vi "SolarPanelSoftware_testeDigiRead.vi"() -> ()   [LabVIEW 2021]
uses:
  <vilib>/MakerHub/LINX/Public/Peripherals/Analog/Analog Read N Chans.vi
  <vilib>/MakerHub/LINX/Private/Local IO/LinxAnalogRead.vi
  <vilib>/MakerHub/LINX/Public/Utilities/Check Channel.vi
  <vilib>/MakerHub/LINX/Public/Utilities/Open Serial.vi
  <vilib>/MakerHub/LINX/Private/Utilties/Generate Error.vi
  <vilib>/MakerHub/LINX/Public/Sensors/Motion/Servo/Servo Open N Channels.vi
  <vilib>/MakerHub/LINX/Public/Sensors/Motion/Servo/Servo Set Pulse Width N Channels.vi
  <vilib>/MakerHub/LINX/Public/Sensors/Motion/Servo/Servo Close N Channels.vi
  <vilib>/MakerHub/LINX/LMH-LINX.lvlib
  <vilib>/MakerHub/LINX/Public/Sensors/Motion/Servo/Servo.lvlib
panel:
  in  "Start Button":bool
  out "BAIXO > CIMA":bool
  out "CIMA > BAIXO":bool
  out "DIR > ESQ":bool
  out "ESQ > DIR":bool
  in  "Servo Channels":i32[](array[numeric])=[9, 110]
  out "Angle Y":dbl
  in  "Threshold":dbl min=0.0 max=2.0 step=0.1
  out "Angle X":dbl
  out "Waveform Chart":T1(graph)
  out "Voltages":dbl[](array[numeric])
  in  "AI Channel(s)":u8[](array[numeric])
  in  "Stop Button":bool
  out "Loop Rate (Hz)":u32
  in  "Serial Port":refnum<visa-resource-name>
  out "ON":bool
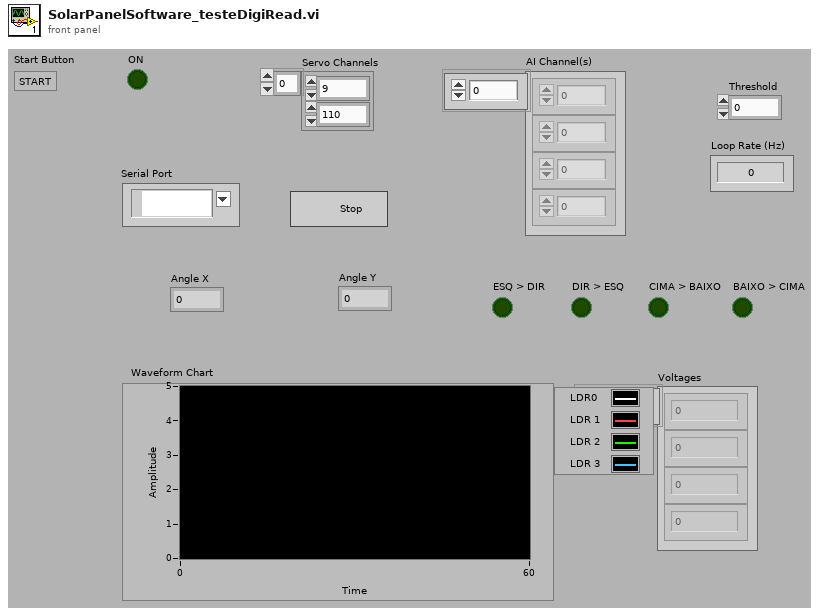
[diagram p1: front panel]
types:
  T1 = cluster{"Voltages[0]":dbl, "Voltages[1]":dbl, "Voltages[2]":dbl, "Voltages[3]":dbl, "Voltages[4]":dbl, "Voltages[5]":dbl, "Voltages[6]":dbl, "Voltages[7]":dbl, "Voltages[8]":dbl}
  T2 = typedef "LMH-LINX.lvlib/LINX Ref.ctl" = cluster{"IO":T3, "Interface":T4, "LINX Device Config":T5}
  T3 = typedef "LMH-LINX.lvlib/Platform.ctl" = enum16{"Remote", "Local"}
  T4 = typedef "LMH-LINX.lvlib/Interface.ctl" = enum16{"Serial", "TCP"}
  T5 = typedef "LMH-LINX.lvlib/Device.lvlib/LINX Device Config.ctl" = cluster{"Interface":T4, "COM Port":refnum<visa-resource-name>, "TCP Configuration":T6, "Device Family":u8, "Device ID":u8, "Device Name":string, "TCP Ref":refnum<k5>, "Channels":T7}
  T6 = typedef "LMH-LINX.lvlib/Device.lvlib/TCP Config.ctl" = cluster{"IP Address":string, "Port":u16}
  T7 = typedef "LMH-LINX.lvlib/Channels.ctl" = cluster{"DI":u8[], "DO":u8[], "AI":u8[], "AO":u8[], "PWM":u8[], "QE":u8[], "UART":u8[], "I2C 2":u8[], "SPI":u8[], "CAN":u8[], "Servo":u8[], "AI Ref (V)":dbl, "AI Resolution (Bits)":u8, "AO Ref (V)":dbl, "AO Resolution (Bits)":u8}
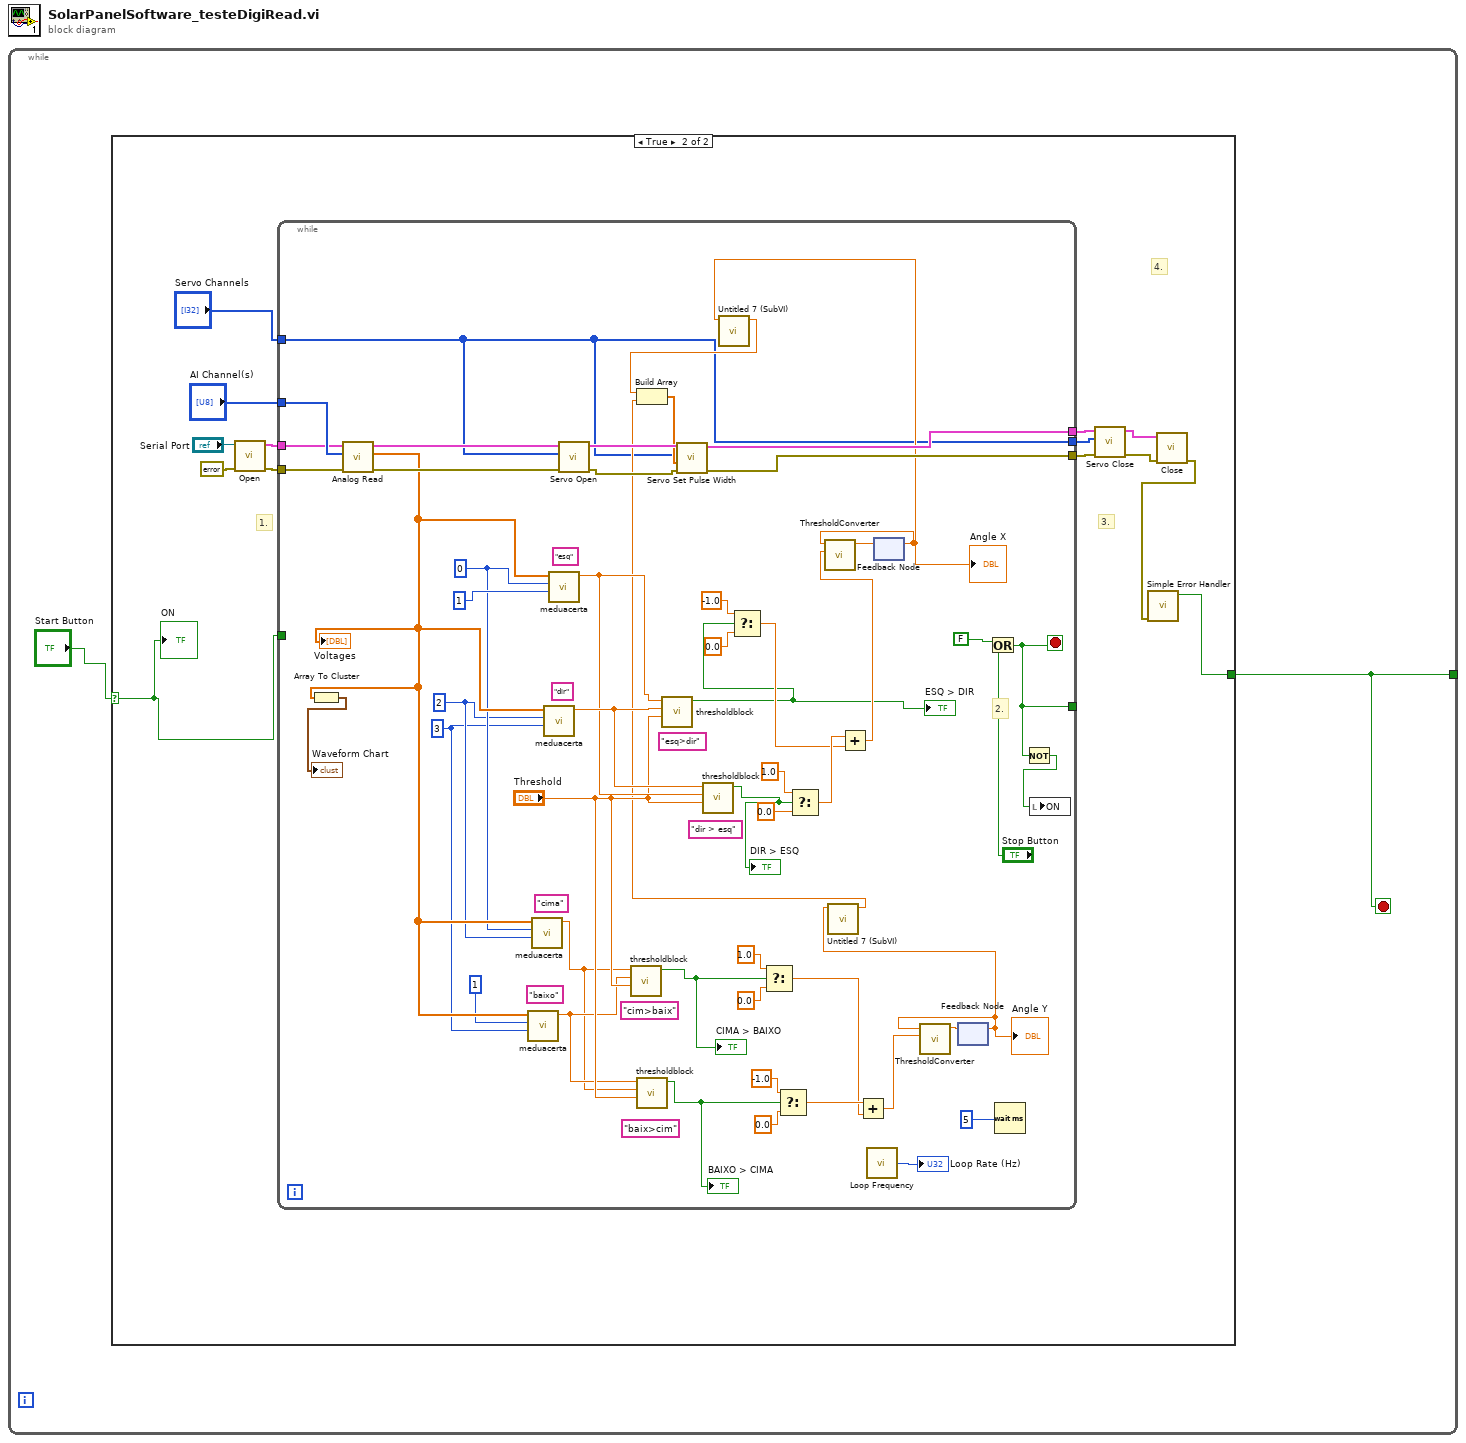
[diagram p0: block diagram]
diagram:
  n1 = while {
    tunnel: [w2] -> _
    stop <- w2 stop-if-true
    n2 = case shown="True" "Start Button" {
      selector: "Start Button" -> [w3 w6]
      tunnel: [w3 w5] -> w2
      frame False {
      }
      frame True {
        # "4."
        # "3."
        # "1."
        n3 = call-poly <vilib>:"Open.vi"("Error In"=errorcluster {"status"=FALSE, "code"=0, "source"=""}, "Serial Port"="Serial Port") -> ("Error Out"=w7:errorcluster, "LINX Resource"=w15:T2)  [unwired: 7 in, 1 out]
        n4 = while {
          tunnel: w15 -> [w66]
          tunnel: "AI Channel(s)" -> [w68]
          tunnel: [w19] -> _
          tunnel: "Servo Channels" -> [w20]
          tunnel: [w61] -> w13
          tunnel: [w60] -> w12
          tunnel: w7 -> [w58]
          tunnel: w6 -> [_]
          tunnel: [w20] -> w4
          stop <- w19 stop-if-true
          (unwired) "baix>cim" ("String")
          (unwired) "cim>baix" ("String")
          (unwired) "esq>dir" ("String")
          (unwired) "dir > esq" ("String")
          (unwired) "dir" ("String")
          (unwired) "esq" ("String")
          (unwired) "cima" ("String")
          (unwired) "baixo" ("String")
          w47 = 3 ("index")
          w49 = 2 ("index")
          w50 = 0 ("index")
          # "2."
          n5 = call-poly <vilib>:"Analog Read.vi"("Error In"=w58, "AI Channel(s)"=w68, "LINX Resource"=w66) -> ("Error Out"=w64:errorcluster, "Voltages"=w52:dbl[], "LINX Resource"=w65:T2)  [unwired: 5 in, 1 out]
          "Voltages" <- w52
          n6 = Array To Cluster(array=w52) -> (cluster=→"Waveform Chart":T1)
          n7 = call "meduacerta.vi"("index 1"=w47, "index 0"=1 ("index"), "Array"=w52) -> ("Média"=w36:dbl)  [unwired: 8 in]
          n8 = call "meduacerta.vi"("index 1"=w49, "index 0"=w50, "Array"=w52) -> ("Média"=w35:dbl)  [unwired: 8 in]
          n9 = call "meduacerta.vi"("index 1"=w47, "index 0"=w49, "Array"=w52) -> ("Média"=w46:dbl)  [unwired: 8 in]
          n10 = call "meduacerta.vi"("index 1"=1 ("index"), "index 0"=w50, "Array"=w52) -> ("Média"=w45:dbl)  [unwired: 8 in]
          n11 = call-poly <vilib>:"Servo Open.vi"("Error In"=w64, "Servo Channels"=w20, "LINX Resource"=w65) -> ("Error Out"=w63:errorcluster, "LINX Resource"=w62:T2)  [unwired: 7 in]
          n12 = call "thresholdblock.vi"("Threshold"="Threshold", "Média 2"=w36, "Média 1"=w35) -> ("Boolean"=w22:bool)  [unwired: 8 in]
          "CIMA > BAIXO" <- w22
          n13 = call "thresholdblock.vi"("Threshold"="Threshold", "Média 2"=w35, "Média 1"=w36) -> ("Boolean"=w21:bool)  [unwired: 8 in]
          "BAIXO > CIMA" <- w21
          n14 = call "thresholdblock.vi"("Threshold"="Threshold", "Média 2"=w46, "Média 1"=w45) -> ("Boolean"=w24:bool)  [unwired: 8 in]
          "ESQ > DIR" <- w24
          n15 = call "thresholdblock.vi"("Threshold"="Threshold", "Média 2"=w45, "Média 1"=w46) -> ("Boolean"=w23:bool)  [unwired: 8 in]
          "DIR > ESQ" <- w23
          n16 = Select(t=-1.0, s=w24, f=0.0) -> (s? t:f=w41:dbl)
          n17 = Select(t=1.0, s=w22, f=0.0) -> (s? t:f=w31:dbl)
          n18 = Select(t=-1.0, s=w21, f=0.0) -> (s? t:f=w32:dbl)
          n19 = Select(t=1.0, s=w23, f=0.0) -> (s? t:f=w42:dbl)
          n20 = Add(x=w42, y=w41) -> (x+y=w40:dbl)
          n21 = Add(x=w32, y=w31) -> (x+y=w29:dbl)
          n22 = call <vilib>:"Loop Frequency.vi"() -> ("Loop Rate (Hz)"=→"Loop Rate (Hz)":u32)
          n23 = feedback #1() -> (w53:dbl)  [unwired: 1 in]
          "Angle X" <- w53
          n24 = call "Untitled 7 (SubVI).vi"("Input"=w53) -> ("Numeric"=w27:dbl)  [unwired: 10 in]
          n25 = call "ThresholdConverter.vi"("Input1"=w40, "Input2"=w53) -> ("Out"=w54:dbl)  [unwired: 9 in]
          n26 = feedback-in #1(w54) -> ()
          n27 = feedback #2() -> (w28:dbl)  [unwired: 1 in]
          "Angle Y" <- w28
          n28 = call "Untitled 7 (SubVI).vi"("Input"=w28) -> ("Numeric"=w26:dbl)  [unwired: 10 in]
          n29 = Build Array(w27, w26) -> (w25:dbl[])
          n30 = call-poly <vilib>:"Servo Set Pulse Width.vi"("Error In"=w63, "Pulse Widths (uS)"=w25, "Servo Channels"=w20, "LINX Resource"=w62) -> ("Error Out"=w60:errorcluster, "LINX Resource"=w61:T2)  [unwired: 6 in]
          n31 = call "ThresholdConverter.vi"("Input1"=w29, "Input2"=w28) -> ("Out"=w30:dbl)  [unwired: 9 in]
          n32 = feedback-in #2(w30) -> ()
          n33 = Or(x=FALSE, y="Stop Button") -> (x .or. y?=w19:bool)
          n34 = Wait (ms)(milliseconds to wait=u32 5) -> ()  [unwired: 1 out]
          n35 = Not(x=w19) -> (.not. x?=w18:bool)
          n36 = local write "ON"(w18) -> ()
        }
        n37 = call-poly <vilib>:"Servo Close.vi"("Error In"=w12, "Servo Channels"=w4, "LINX Resource"=w13) -> ("Error Out"=w10:errorcluster, "LINX Resource"=w11:T2)  [unwired: 7 in]
        n38 = call <vilib>:"Close.vi"("Error In"=w10, "LINX Resource"=w11) -> ("Error Out"=w9:errorcluster)  [unwired: 9 in]
        n39 = call <vilib>:"Simple Error Handler.vi"("error in (no error)"=w9) -> ("error?"=w5:bool)  [unwired: 4 in, 4 out]
        "ON" <- w6
      }
    }
  }
